vi "Release Msg Q.vi"(11 "Msg Queue in":refnum<class "Msg Q.lvclass">) -> (0 "error out":errorcluster, 2 "Remaining Elements":refnum<class "Msg.lvclass">[](array[class]))   [LabVIEW 2021, in "LVCAM.lvlib" / "Msg Q.lvclass"]
uses:
  Msg Q.lvclass
  Msg/Msg.lvclass
  Msg Q.lvclass/Msg Q.ctl
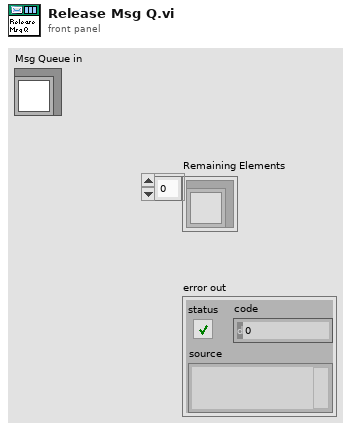
[diagram p1: front panel]
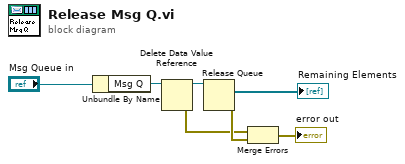
[diagram p0: block diagram]
diagram:
  n1 = Unbundle By Name("Msg Queue in") -> ("Msg Q"=w7:refnum<data-value>)
  n2 = Delete Data Value Reference(data value reference=w7) -> (data value=w6:refnum<queue>, error out=w3:errorcluster)  [unwired: 1 in]
  n3 = Release Queue(queue=w6) -> (remaining elements=→"Remaining Elements":refnum<class "Msg.lvclass">[], error out=w4:errorcluster)  [unwired: 2 in, 1 out]
  n4 = Merge Errors(w3, w4) -> (→"error out":errorcluster)
